vi "Main.vi"() -> ()   [LabVIEW 2017]
uses:
  <vilib>/FPGAPlugInAG/PCIe-7852R/niLvFpga_Open_PCIe-7852R.vi
  <vilib>/FPGAPlugInAG/PCIe-7852R/niLvFpga_Abort_PCIe-7852R.vi
  <vilib>/FPGAPlugInAG/PCIe-7852R/niLvFpga_Reset_PCIe-7852R.vi
  <vilib>/rvi/interface/common/niFpgaWaitOnOcc.vi
  <vilib>/Utility/error.llb/Error Cluster From Error Code.vi
  <vilib>/FPGAPlugInAG/PCIe-7852R/niLvFpga_Run_PCIe-7852R.vi
  <vilib>/rvi/errors/niLvFpgaAdjustHostInterfaceError.vi
  <vilib>/FPGAPlugInAG/PCIe-7852R/niLvFpga_Close_PCIe-7852R.vi
  <vilib>/rvi/interface/nirviOpenFPGA/nirviOpenFPGA.xnode
  FPGA Bitfiles/Galvo Calibrator - Bitfiles.lvbitx
  <vilib>/rvi/interface/nirviMethod/nirviMethod.xnode
  <vilib>/rvi/interface/nirviReadWriteControl/nirviReadWriteControl.xnode
  <vilib>/rvi/interface/nirviCloseFPGA/nirviCloseFPGA.xnode
  NiFpgaLv.dll
  <vilib>/rvi/errors/niLvFpgaMergeErrorWithErrorCode.vi
  <vilib>/FPGAPlugInAG/PCIe-7852R/niLvFpga_ConfigureFifo_PCIe-7852R.vi
  <vilib>/FPGAPlugInAG/PCIe-7852R/niLvFpga_StartFifo_PCIe-7852R.vi
  <vilib>/FPGAPlugInAG/PCIe-7852R/niLvFpga_ReadFifo_PCIe-7852R.vi
  <vilib>/FPGAPlugInAG/PCIe-7852R/niLvFpga_StopFifo_PCIe-7852R.vi
panel:
  in  "Z Phase Shift (Deg)":dbl caption="Phase Shift (Deg)"
  in  "Z AO Amplitude (V)":dbl=5.0 caption="AO Amplitude (V)" min=0.0 max=10.0
  in  "Z Frequency (Hz)":dbl=5.0 caption="Frequency (Hz)" min=0.0 max=1000.0 step=1.0
  out "AO DMA Overflow":bool
  out "AO":dbl[][](graph)
  in  "X Phase Shift (Deg)":dbl caption="Phase Shift (Deg)"
  in  "Sync DDS":bool
  in  "X AO Amplitude (V)":dbl=5.0 caption="AO Amplitude (V)" min=0.0 max=10.0
  in  "X Frequency (Hz)":dbl=5.0 caption="Frequency (Hz)" min=0.0 max=1000.0 step=1.0
  in  "AO Update Freq (Hz)":dbl=100000.0 format="%#_6p"
  # "X Galvo"
  # "Z Galvo"
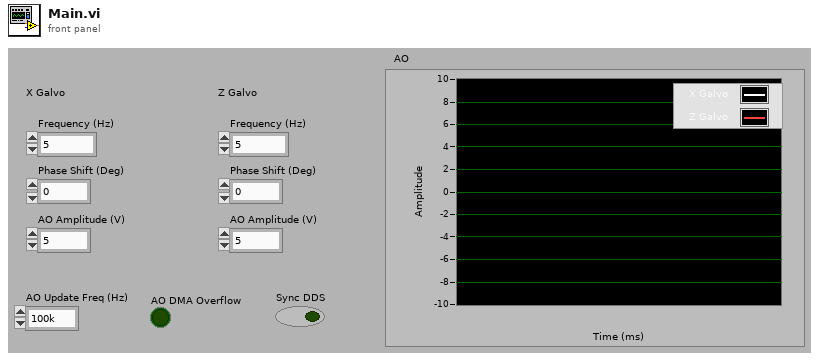
[diagram p1: front panel]
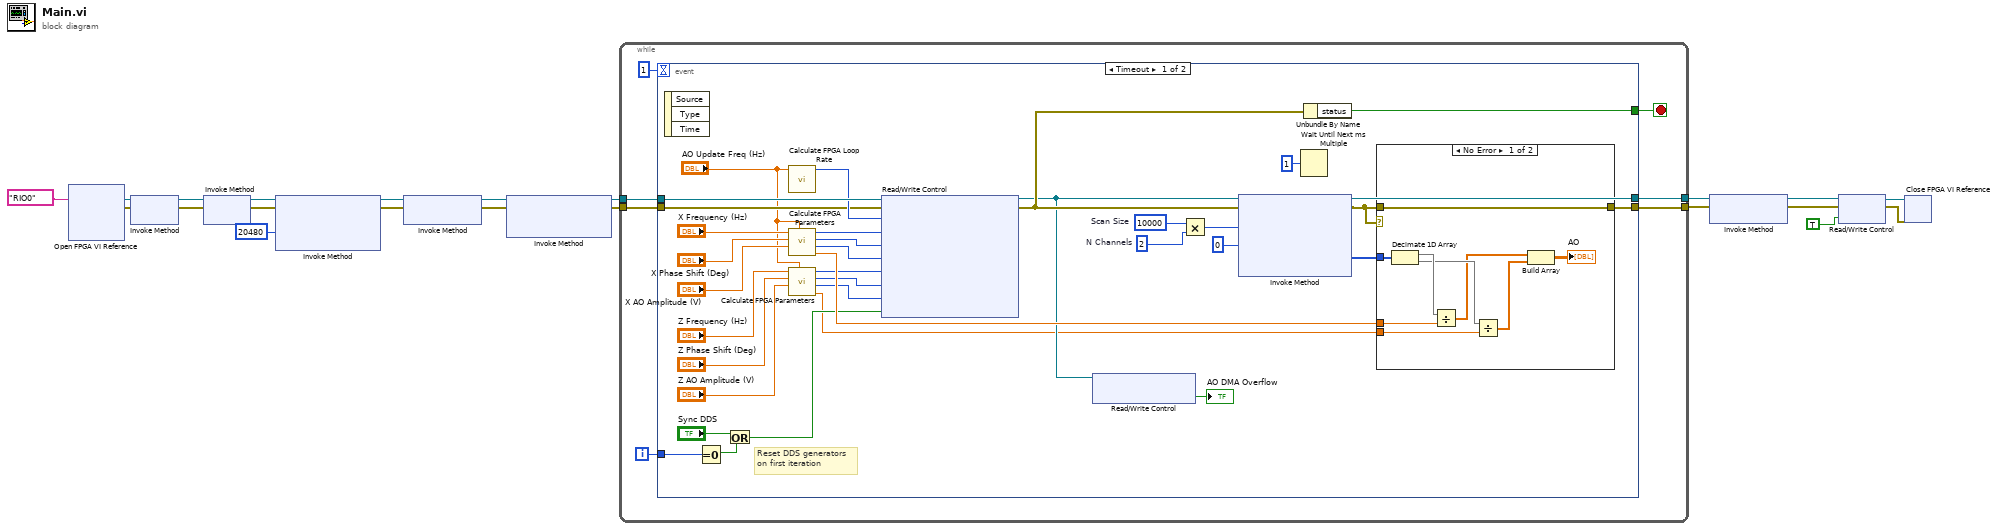
[diagram p0: block diagram]
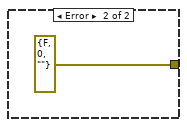
[diagram p2: hidden frame]
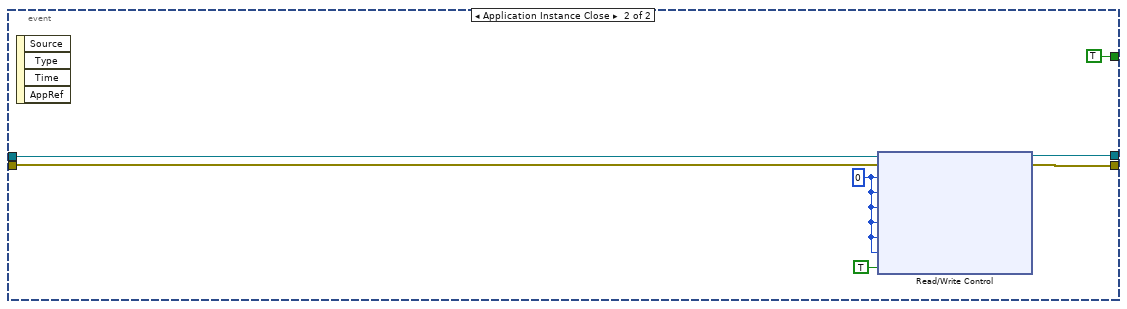
[diagram p3: hidden frame]
diagram:
  n1 = xnode "Open FPGA VI Reference"("resource name"=tag "RIO0") -> ("FPGA VI Reference Out"=w21:refnum<k20>, "error out"=w20:errorcluster)  [unwired: 1 in]
  n2 = xnode "Invoke Method"("FPGA VI Reference In"=w21, "error in"=w20) -> ("FPGA VI Reference Out"=w19:refnum<k20>, "error out"=w18:errorcluster)
  n3 = xnode "Invoke Method"("FPGA VI Reference In"=w19, "error in"=w18) -> ("FPGA VI Reference Out"=w15:refnum<k20>, "error out"=w3:errorcluster)
  n4 = xnode "Invoke Method"("FPGA VI Reference In"=w15, "error in"=w3, "Requested Depth"=u32 20480) -> ("FPGA VI Reference Out"=w4:refnum<k20>, "error out"=w2:errorcluster)  [unwired: 1 out]
  n5 = xnode "Invoke Method"("FPGA VI Reference In"=w4, "error in"=w2) -> ("FPGA VI Reference Out"=w9:refnum<k20>, "error out"=w8:errorcluster)
  n6 = xnode "Invoke Method"("FPGA VI Reference In"=w9, "error in"=w8) -> ("FPGA VI Reference Out"=w17:refnum<k20>, "error out"=w16:errorcluster)  [unwired: 1 in]
  n7 = while {
    tunnel: w17 -> [w28]
    tunnel: w16 -> [w26]
    tunnel: [w24] -> w6
    tunnel: [w25] -> w14
    i -> [w27]
    stop <- w23 stop-if-true
    n8 = event shown="[0] Timeout" {
      selector: _ -> [_ _]
      dyn-events: _ -> [_ _]
      timeout: 1 -> [_ _]
      tunnel: w28 -> [w63 w76]
      tunnel: w27 -> [w53 _]
      tunnel: w26 -> [w51 w77]
      tunnel: [w50 w79] -> w25
      tunnel: [w47 w78] -> w24
      tunnel: [w29 TRUE ("status")] -> w23
      event Timeout {
        w39 = u32 2  # N Channels
        w40 = u32 10000  # Scan Size
        # "Reset DDS generators\non first iteration"
        n9 = event-data() -> ()  [unwired: 1 in, 3 out]
        n10 = Equal To 0?(x=w53) -> (x = 0?=w52:bool)
        n11 = Or(x="Sync DDS", y=w52) -> (x .or. y?=w38:bool)
        n12 = call "Calculate FPGA Loop Rate.vi"("Loop Frequency (Hz)"="AO Update Freq (Hz)") -> ("Loop  Rate (ticks)"=w59:u32)  [unwired: 10 in]
        n13 = call "Calculate FPGA Parameters.vi"("Loop Rate (Hz)"="AO Update Freq (Hz)", "Signal Amplitude (V)"="X AO Amplitude (V)", "Phase Shift (Deg)"="X Phase Shift (Deg)", "DDS Signal Frequency (Hz)"="X Frequency (Hz)") -> ("Scaling Ratio"=w45:dbl, "AO Amplitude"=w55:u16, "Phase Shift"=w56:u32, "Accumulator Increment"=w60:u32)  [unwired: 4 in]
        n14 = call "Calculate FPGA Parameters.vi"("Loop Rate (Hz)"="AO Update Freq (Hz)", "Signal Amplitude (V)"="Z AO Amplitude (V)", "Phase Shift (Deg)"="Z Phase Shift (Deg)", "DDS Signal Frequency (Hz)"="Z Frequency (Hz)") -> ("Scaling Ratio"=w30:dbl, "AO Amplitude"=w35:u16, "Phase Shift"=w36:u32, "Accumulator Increment"=w37:u32)  [unwired: 4 in]
        n15 = xnode "Read/Write Control"("FPGA VI Reference In"=w63, "error in"=w51, "Update Rate (ticks)"=w59, "X Accumulator Increment"=w60, "X Phase Shift"=w56, "X Signal Amplitude"=w55, "Z Accumulator Increment"=w37, "Z Phase Shift"=w36, "Z Signal Amplitude"=w35, "Reset Accumulator"=w38) -> ("FPGA VI Reference Out"=w44:refnum<k20>, "error out"=w49:errorcluster)
        n16 = xnode "Read/Write Control"("FPGA VI Reference In"=w44) -> ("AO DMA Overflow"=→"AO DMA Overflow":bool)  [unwired: 1 in, 2 out]
        n17 = Multiply(x=w40, y=w39) -> (x*y=w41:u32)
        n18 = xnode "Invoke Method"("FPGA VI Reference In"=w44, "error in"=w49, "Number of Elements"=w41, "Timeout (ms)"=0) -> ("FPGA VI Reference Out"=w50:refnum<k20>, "error out"=w42:errorcluster, "Data"=w46:i16[])  [unwired: 1 out]
        n19 = Wait Until Next ms Multiple(millisecond multiple=u32 1) -> ()  [unwired: 1 out]
        n20 = Unbundle By Name(w49) -> ("status"=w29:bool)
        n21 = case shown="No Error" w42 {
          tunnel: w42 -> [w72 _]
          tunnel: [w72 errorcluster {"status"=FALSE, "code"=0, "source"=""} ("error out")] -> w47
          tunnel: w46 -> [w71 _]
          tunnel: w45 -> [w70 _]
          tunnel: w30 -> [w68 _]
          frame No Error {
            n22 = Decimate 1D Array(w71) -> (w69:i16[], w67:i16[])
            n23 = Divide(x=w69, y=w70) -> (x/y=w66:dbl[])
            n24 = Divide(x=w67, y=w68) -> (x/y=w65:dbl[])
            n25 = Build Array(w66, w65) -> (→"AO":dbl[][])
          }
          frame Error {
          }
        }
      }
      event Application Instance Close {
        w75 = u32 0 ("X Accumulator Increment")
        n26 = event-data() -> ()  [unwired: 1 in, 4 out]
        n27 = xnode "Read/Write Control"("FPGA VI Reference In"=w76, "error in"=w77, "X Accumulator Increment"=w75, "X Phase Shift"=w75, "X Signal Amplitude"=w75, "Z Accumulator Increment"=w75, "Z Phase Shift"=w75, "Z Signal Amplitude"=w75, "Reset Accumulator"=TRUE) -> ("FPGA VI Reference Out"=w79:refnum<k20>, "error out"=w78:errorcluster)
      }
    }
  }
  n28 = xnode "Invoke Method"("FPGA VI Reference In"=w14, "error in"=w6) -> ("FPGA VI Reference Out"=w7:refnum<k20>, "error out"=w5:errorcluster)
  n29 = xnode "Read/Write Control"("FPGA VI Reference In"=w7, "error in"=w5, "Stop"=TRUE) -> ("FPGA VI Reference Out"=w11:refnum<k20>, "error out"=w12:errorcluster)
  n30 = xnode "Close FPGA VI Reference"("FPGA VI Reference In"=w11, "error in"=w12) -> ()  [unwired: 1 out]
